vi "controlNav.vi"() -> ()   [LabVIEW 2014]
uses:
  <vilib>/LVH/AR Drone Toolkit/AR Drone.lvlib
  <vilib>/Utility/inputDevices.llb/closeJoystick.vi
  <vilib>/LVH/AR Drone Toolkit/Decode NavData/Typedefs/NavData Demo.ctl
panel:
  out "Gamepad Output 2":T1
  out "NavData Out":T2
  out "Battery Remaining":dbl(slide) scale=0.0..100.0
  in  "stop":bool
  out "Axes Output":T3 {"Vertical Speed" scale=-1.0..1.0; "Yaw Speed" scale=-1.0..1.0; "Pitch" scale=-1.0..1.0; "Roll" scale=-1.0..1.0}
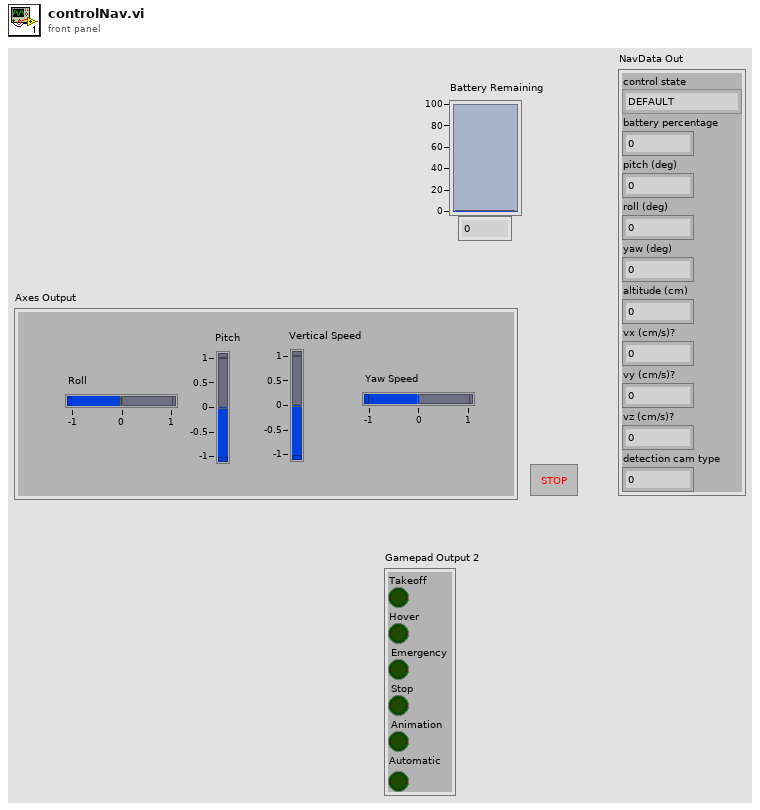
[diagram p1: front panel]
types:
  T1 = cluster{"Takeoff":bool, "Hover":bool, "Emergency":bool, "Stop":bool, "Animation":bool, "Automatic":bool}
  T2 = typedef "AR Drone.lvlib/NavData Demo.ctl" = cluster{"control state":enum32{"DEFAULT", "INIT", "LANDING", "FLYING", "HOVERING", "TEST", "TRANS_TAKEOFF", "TRANS_GOTOFIX", "TRANS_LANDING"}, "battery percentage":u32, "pitch (deg)":sgl, "roll (deg)":sgl, "yaw (deg)":sgl, "altitude (cm)":u32, "vx (cm/s)?":sgl, "vy (cm/s)?":sgl, "vz (cm/s)?":sgl, "detection cam type":u32}
  T3 = cluster{"Roll":dbl, "Pitch":dbl, "Vertical Speed":dbl, "Yaw Speed":dbl}
  T4 = typedef "AR Drone.lvlib/AR Drone Resource.ctl" = cluster{"UDP Control Connection":refnum<k16>, "UDP NavData Connection":refnum<k16>, "UDP Video Connection (Drone 1.0)":refnum<k16>, "TCP Video Connection (Drone 2.0)":refnum<k5>, "TCP Control Port Connection":refnum<k5>, "Drone IP address":string, "Drone Command Port":u16, "Drone NavData Port":u16, "Drone Vid Stream Port":u16, "Drone TCP Control Port":u16, "Home IP address":string, "Home Command Port":u16, "Home NavData Port":u16, "Home Vid Stream Port":u16, "Drone Version":i32}
  T5 = cluster{"Roll":sgl, "Pitch":sgl, "Vertical Speed":sgl, "Yaw Speed":sgl}
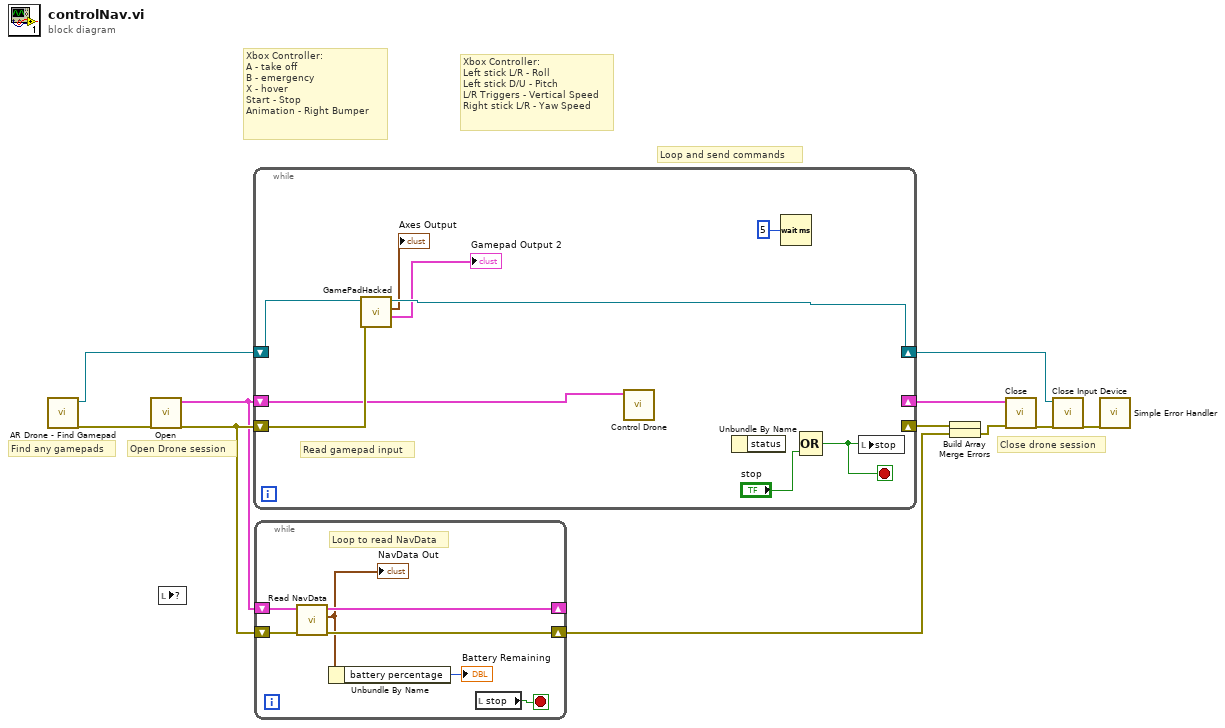
[diagram p0: block diagram]
diagram:
  # "Loop and send commands"
  # "Close drone session"
  # "Open Drone session"
  # "Find any gamepads"
  # "Xbox Controller:\nLeft stick L/R - Roll\nLeft stick D/U - Pitch\nL/R Triggers - Vertical Speed\nRight stick L/R - Yaw Speed"
  # "Xbox Controller:\nA - take off\nB - emergency\nX - hover\nStart - Stop\nAnimation - Right Bumper"
  n1 = call "AR Drone - Find Gamepad.vi"() -> ("error out"=w7:errorcluster, "Refnum out"=w8:refnum<k1>)  [unwired: 10 in]
  n2 = call <vilib>:"Open.vi"("error in (no error)"=w7) -> ("error out"=w3:errorcluster, "AR Drone Resource"=w1:T4)  [unwired: 9 in]
  n3 = local read item#-1() -> ()  [unwired: 1 in]
  n4 = while {
    shift-right: [_] -> w12
    shift-left: w1 -> [w13]
    shift-right: [_] -> w5
    shift-left: w3 -> [w16]
    shift-right: [w18] -> w11
    shift-left: w8 -> [w17]
    stop <- w19 stop-if-true
    # "Read gamepad input"
    n5 = call "GamePadHacked.vi"("error in (no error)"=w16, "Refnum in"=w17) -> ("Gamepad Output"=→"Gamepad Output 2":T1, "Control Cluster"=→"Axes Output":T5, "Refnum out"=w18:refnum<k1>)  [unwired: 6 in, 1 out]
    n6 = call <vilib>:"Control Drone.vi"("AR Drone Resource"=w13) -> ()  [unwired: 9 in, 2 out]
    n7 = Unbundle By Name() -> ()  [unwired: 1 in, 1 out]
    n8 = Wait (ms)(milliseconds to wait=u32 5) -> ()  [unwired: 1 out]
    n9 = Compound Arithmetic op=OR("stop") -> (w19:bool)  [unwired: 2 in]
    n10 = local write "stop"(w19) -> ()
  }
  n11 = while {
    shift-right: [w27] -> _
    shift-left: w1 -> [w28]
    shift-right: [w25] -> w4
    shift-left: w3 -> [w26]
    stop <- w22 stop-if-true
    # "Loop to read NavData"
    n12 = call <vilib>:"Read NavData.vi"("error in (no error)"=w26, "AR Drone Resource"=w28) -> ("error out"=w25:errorcluster, "NavData Out"=w24:T2, "AR Drone Resource Out"=w27:T4)  [unwired: 7 in]
    "NavData Out" <- w24
    n13 = Unbundle By Name(w24) -> ("battery percentage"=→"Battery Remaining":u32)
    n14 = local read "stop"() -> (w22:bool)
  }
  n15 = Build Array(w5, w4) -> (w2:errorcluster[])
  n16 = Merge Errors(w2) -> (w6:errorcluster)
  n17 = call <vilib>:"Close.vi"("error in (no error)"=w6, "AR Drone Resource"=w12) -> ("error out"=w10:errorcluster)  [unwired: 9 in]
  n18 = call-poly <vilib>:"Close Input Device.vi"("error in (no error)"=w10, "device ID"=w11) -> ("error out"=w9:errorcluster)  [unwired: 8 in]
  n19 = call <vilib>:"Simple Error Handler.vi"("error in (no error)"=w9) -> ()  [unwired: 4 in, 5 out]
